vi "chkIfSecMeetWithVarRuleInC.vi"(11 "section":string) -> (3 "meetWithVarRuleInC?":bool)   [LabVIEW 2010]
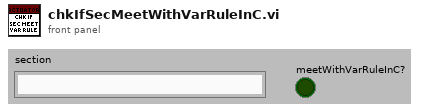
[diagram p1: front panel]
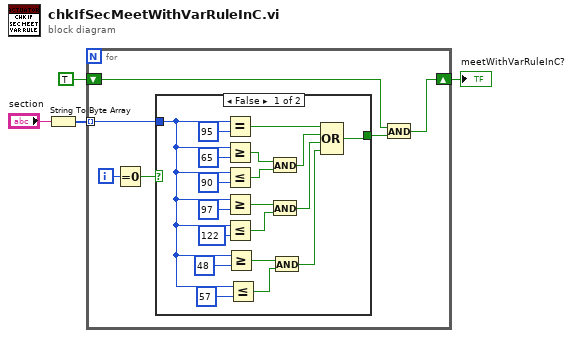
[diagram p0: block diagram]
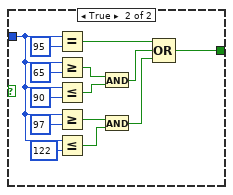
[diagram p2: hidden frame]
diagram:
  n1 = String To Byte Array(string="section") -> (unsigned byte array=w3:u8[])
  n2 = for {
    tunnel: w3 -> [w8] mode=indexing
    shift-right: [w5] -> w1
    shift-left: TRUE -> [w6]
    i -> [w10]
    n3 = Equal To 0?(x=w10) -> (x = 0?=w9:bool)
    n4 = case shown="False" w9 {
      tunnel: w8 -> [w15 w36]
      tunnel: [w17 w30] -> w7
      frame False {
        n5 = Equal?(x=w15, y=u8 95) -> (x = y?=w28:bool)
        n6 = Greater Or Equal?(x=w15, y=u8 65) -> (x >= y?=w25:bool)
        n7 = Less Or Equal?(x=w15, y=u8 90) -> (x <= y?=w24:bool)
        n8 = Greater Or Equal?(x=w15, y=u8 97) -> (x >= y?=w21:bool)
        n9 = Less Or Equal?(x=w15, y=u8 122) -> (x <= y?=w20:bool)
        n10 = Greater Or Equal?(x=w15, y=u8 48) -> (x >= y?=w13:bool)
        n11 = Less Or Equal?(x=w15, y=u8 57) -> (x <= y?=w12:bool)
        n12 = And(x=w25, y=w24) -> (x .and. y?=w19:bool)
        n13 = And(x=w21, y=w20) -> (x .and. y?=w18:bool)
        n14 = And(x=w13, y=w12) -> (x .and. y?=w11:bool)
        n15 = Compound Arithmetic op=OR(w28, w19, w18, w11) -> (w17:bool)
      }
      frame True {
        n16 = Equal?(x=w36, y=u8 95) -> (x = y?=w42:bool)
        n17 = Greater Or Equal?(x=w36, y=u8 65) -> (x >= y?=w39:bool)
        n18 = Less Or Equal?(x=w36, y=u8 90) -> (x <= y?=w38:bool)
        n19 = Greater Or Equal?(x=w36, y=u8 97) -> (x >= y?=w34:bool)
        n20 = Less Or Equal?(x=w36, y=u8 122) -> (x <= y?=w33:bool)
        n21 = And(x=w39, y=w38) -> (x .and. y?=w32:bool)
        n22 = And(x=w34, y=w33) -> (x .and. y?=w31:bool)
        n23 = Compound Arithmetic op=OR(w42, w32, w31) -> (w30:bool)
      }
    }
    n24 = And(x=w6, y=w7) -> (x .and. y?=w5:bool)
  }
  "meetWithVarRuleInC?" <- w1
